vi "Write XNET Array.vi"(8 "error in (no error)":errorcluster, 10 "XNET Array":T1[](array[typedef]) {"payload" format="%x"; "timestamp" format="%<%.7X\n%x>T"; "type" items=["CAN Data"=0, "CAN Remote"=1, "CAN Bus Error"=2, "CAN 2.0 Data"=8, "CAN FD Data"=16, "CAN FD+BRS Data"=24, "J1939 Data"=192, "Delay"=224, "Log Trigger"=225, "Start Trigger"=226]; "identifier" format="%x"}, 11 "XNET Data in":refnum<class "XNET Data.lvclass">) -> (0 "error out":errorcluster, 3 "XNET Data out":refnum<class "XNET Data.lvclass">)   [LabVIEW 2021, in "BS120x Driver.lvlib" / "Data Classes.lvlib" / "XNET Data.lvclass"]
uses:
  XNET Data.lvclass
  <vilib>/xnet/xnet.llb/XNET Frame CAN.ctl
  <vilib>/xnet/xnet.llb/XNET Frame Type CAN.ctl
  XNET Data.lvclass/XNET Data.ctl
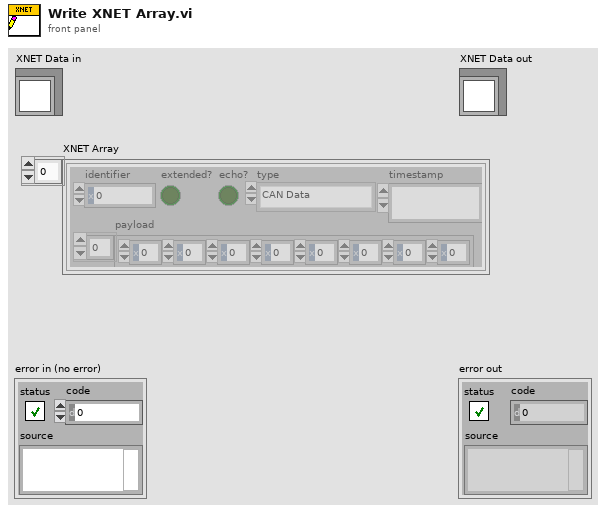
[diagram p1: front panel]
types:
  T1 = typedef "XNET Frame CAN.ctl" = cluster{"timestamp":timestamp, "payload":u8[], "identifier":u32, "type":T2, "extended?":bool, "echo?":bool}
  T2 = typedef "XNET Frame Type CAN.ctl" = u8
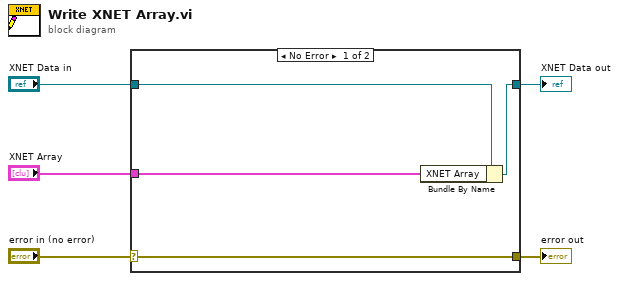
[diagram p0: block diagram]
diagram:
  n1 = case shown="No Error" "error in (no error)" {
    selector: "error in (no error)" -> [w9 w10]
    tunnel: [w9 w10] -> w4
    tunnel: [w7 w11] -> w2
    tunnel: "XNET Data in" -> [w8 w11]
    tunnel: "XNET Array" -> [w6 _]
    frame No Error {
      n2 = Bundle By Name(cluster=w8, "XNET Array"=w6) -> (w7:refnum<class "XNET Data.lvclass">)
    }
    frame Error {
    }
  }
  "error out" <- w4
  "XNET Data out" <- w2
